vi "Omron Serial FINS-Initialize.vi"(8 "error in":errorcluster, 11 "Connection Data In":T3={"VISA Resource Name"="", "Baud Rate"=115200, "Data Bits"=7, "Parity"=0, "Stop Bits"=20, "Wait For Read(ms)"=50} {"Stop Bits" items=["1.0"=10, "1.5"=15, "2.0"=20]; "Parity" items=["None", "Odd", "Even", "Mark", "Space"]}) -> (0 "error out":errorcluster, 3 "Buffer Data":T1={"VISA Resource Name"="", "Wait For Read(ms)"=50, "Command Code"=enum."Memory area read", "Command String"="", "Read Bytes"=0, "Response String"=""})   [LabVIEW 2016]
uses:
  Data Def/Omron Serial FINS-Connection Data.ctl
  Data Def/Omron Serial FINS-Buffer Data.ctl
  Data Def/Omron Serial FINS-Command Code.ctl
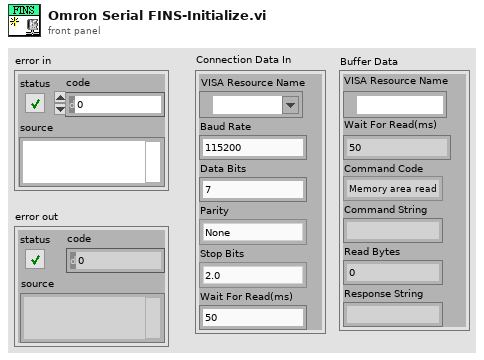
[diagram p1: front panel]
types:
  T1 = typedef "Omron Serial FINS-Buffer Data.ctl" = cluster{"VISA Resource Name":refnum<visa-resource-name>, "Wait For Read(ms)":u32, "Command Code":T2, "Command String":string, "Read Bytes":u32, "Response String":string}
  T2 = typedef "Omron Serial FINS-Command Code.ctl" = enum16{"Memory area read", "Memory area write"}
  T3 = typedef "Omron Serial FINS-Connection Data.ctl" = cluster{"VISA Resource Name":refnum<visa-resource-name>, "Baud Rate":u32, "Data Bits":u16, "Parity":u16, "Stop Bits":u16, "Wait For Read(ms)":u32}
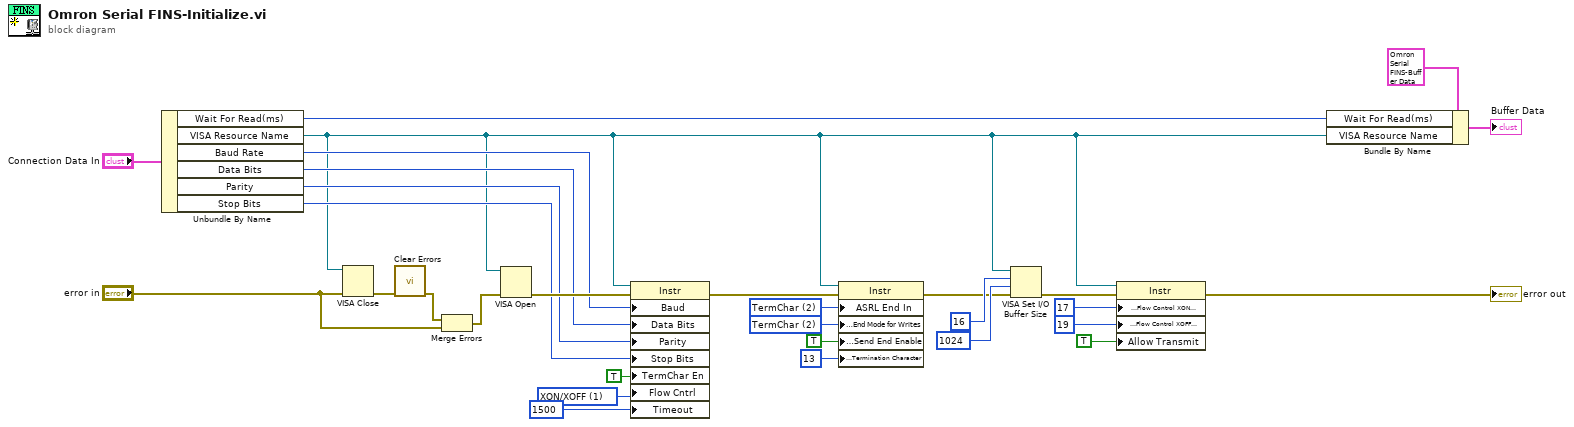
[diagram p0: block diagram]
diagram:
  w3 = u16 2 items=["None", "Last Bit", "TermChar"] ("Serial Settings:End Mode for Reads")
  w4 = u16 2 items=["None", "LastBit", "TermChar", "Break"] ("Serial Settings:Serial End Mode for Writes")
  w19 = u16 1 items=["None", "XON/XOFF", "RTS/CTS", "XON/XOFF & RTS/CTS", "DTR/DSR", "XON/XOFF & DTR/DSR"] ("Serial Settings:Flow Control")
  n1 = Unbundle By Name("Connection Data In") -> ("Wait For Read(ms)"=w12:u32, "VISA Resource Name"=w13:refnum<visa-resource-name>, "Baud Rate"=w24:u32, "Data Bits"=w23:u16, "Parity"=w22:u16, "Stop Bits"=w21:u16)
  n2 = VISA Close(VISA resource name=w13, error in (no error)="error in") -> (error out=w28:errorcluster)
  n3 = call <vilib>:"Clear Errors.vi"("error in (no error)"=w28) -> ("error out"=w27:errorcluster)  [unwired: 5 in, 1 out]
  n4 = Merge Errors(w27, "error in") -> (w26:errorcluster)
  n5 = VISA Open(error in (no error)=w26, VISA resource name=w13) -> (error out=w25:errorcluster)  [unwired: 3 in, 1 out]
  n6 = property class="Instr"(reference=w13, error in=w25, "Baud"=w24, "Data Bits"=w23, "Parity"=w22, "Stop Bits"=w21, "TermChar En"=TRUE ("Message Based Settings:Termination Character Enable"), "Flow Cntrl"=w19, "Timeout"=u32 1500 ("General Settings:Timeout Value")) -> (error out=w18:errorcluster)  [unwired: 1 out]
  n7 = property class="Instr"(reference=w13, error in=w18, "ASRL End In"=w3, "Serial Settings:End Mode for Writes"=w4, "Message Based Settings:Send End Enable"=TRUE ("End write with termination character?"), "Message Based Settings:Termination Character"=u8 13 ("termination char\n(0xA = '\\n' = LF)")) -> (error out=w6:errorcluster)  [unwired: 1 out]
  n8 = VISA Set I/O Buffer Size(VISA resource name=w13, mask (16)=u16 16 ("I/O Receive\nBuffer mask"), size (4096)=u32 1024 ("Input\nbuffer size"), error in (no error)=w6) -> (error out=w8:errorcluster)  [unwired: 1 out]
  n9 = property class="Instr"(reference=w13, error in=w8, "Serial Settings:Flow Control XON Character"=u8 17 ("XON Character"), "Serial Settings:Flow Control XOFF Character"=u8 19 ("XOFF Character"), "Allow Transmit"=TRUE ("Serial Settings:Allow Transmit")) -> (error out=→"error out":errorcluster)  [unwired: 1 out]
  n10 = Bundle By Name(cluster=T1 {"VISA Resource Name"="", "Wait For Read(ms)"=50, "Command Code"=enum."Memory area read", "Command String"="", "Read Bytes"=0, "Response String"=""} ("Buffer Data"), "Wait For Read(ms)"=w12, "VISA Resource Name"=w13) -> (→"Buffer Data":T1)
